vi "Search for Element by Attribute.vi"(8 "Identifying Attribute Value":string, 9 "Identifying Attribute Type":string, 10 "Element Type":string, 11 "XML String":string) -> (0 "Element Tag Out":string, 1 "id":string, 2 "Found?":bool, 3 "XML String Out":string)   [LabVIEW 2019, in "EditSVG.lvclass"]
uses:
  EditSVG.lvclass
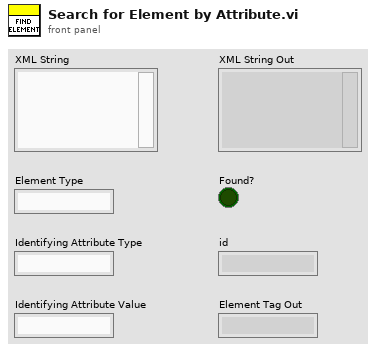
[diagram p1: front panel]
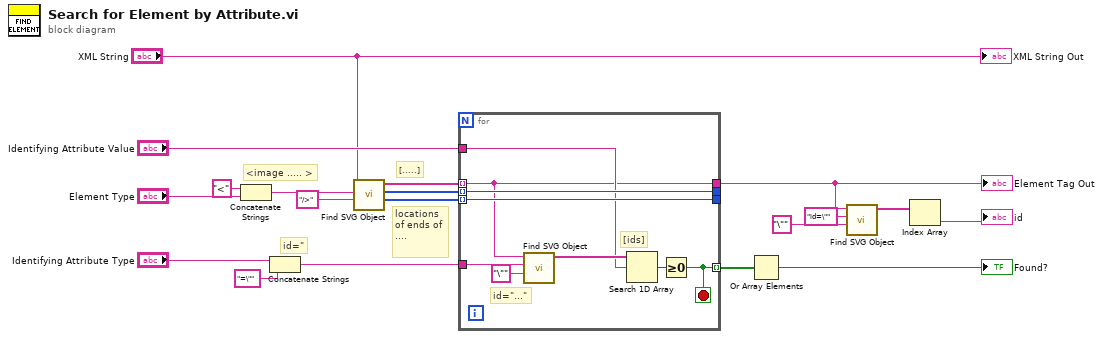
[diagram p0: block diagram]
diagram:
  # "id=\""
  # "locations of ends of ...."
  # "[.....]"
  # "<image ..... >"
  n1 = Concatenate Strings("<" ("string"), "Element Type") -> (w13:string)
  n2 = Concatenate Strings("Identifying Attribute Type", "=\"" ("string")) -> (w16:string)
  n3 = call "Find SVG Object.vi"("Ending Delimiter"="/>", "Beginning Delimiter"=w13, "XML String"="XML String") -> ("Ending Indices"=w15:i32[], "Beginning Indices"=w9:i32[], "Found Values"=w18:string[])  [unwired: 6 in]
  n4 = for {
    tunnel: w18 -> [w20] mode=indexing
    tunnel: w16 -> [w27]
    tunnel: "Identifying Attribute Value" -> [w22]
    tunnel: w15 -> [w26] mode=indexing
    tunnel: [w26] -> _
    tunnel: [w23] -> _
    tunnel: w9 -> [w23] mode=indexing
    tunnel: [w21] -> w8 mode=indexing
    tunnel: [w20] -> w5
    stop <- w21 stop-if-true
    # "id=\"...\""
    # "[ids]"
    n5 = call "Find SVG Object.vi"("Ending Delimiter"="\"", "Beginning Delimiter"=w27, "XML String"=w20) -> ("Found Values"=w25:string[])  [unwired: 6 in, 2 out]
    n6 = Search 1D Array(1D array=w25, element=w22) -> (index of element=w24:i32)  [unwired: 1 in]
    n7 = Greater Or Equal To 0?(x=w24) -> (x >= 0?=w21:bool)
  }
  "Element Tag Out" <- w5
  n8 = Or Array Elements(Boolean array=w8) -> (logical OR=→"Found?":bool)
  n9 = call "Find SVG Object.vi"("Ending Delimiter"="\"", "Beginning Delimiter"="id=\"", "XML String"=w5) -> ("Found Values"=w3:string[])  [unwired: 6 in, 2 out]
  n10 = Index Array(array=w3) -> (element=→"id":string)  [unwired: 1 in]
  "XML String Out" <- "XML String"
